vi "TCP数据转换送显示山推.vi"(1 "原始数据":string) -> (0 "数据提取显示":dbl[](array[numeric]))   [LabVIEW 2016]
panel:
  out "*(类型 *) &x":string
  out "截取数据":string
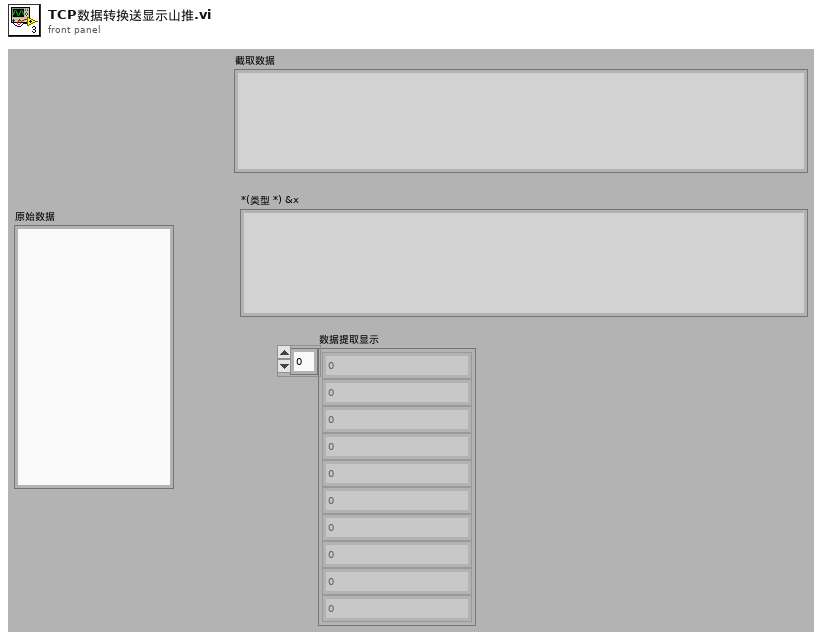
[diagram p1: front panel]
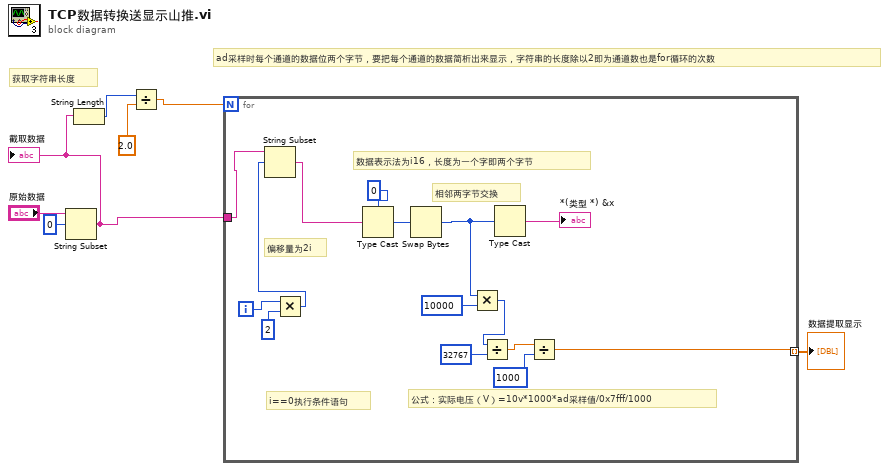
[diagram p0: block diagram]
diagram:
  # "ad采样时每个通道的数据位两个字节，要把每个通道的数据简析出来显示，字符串的长度除以2即为通道数也是for循环的次数"
  # "获取字符串长度"
  n1 = String Subset(string="原始数据", offset (0)=0 ("偏移量(0)")) -> (substring=w5:string)  [unwired: 1 in]
  "截取数据" <- w5
  n2 = String Length(string=w5) -> (length=w3:i32)
  n3 = Divide(x=w3, y=2.0) -> (x/y=w2:dbl)
  n4 = for {
    N: w2 -> [_]
    tunnel: w5 -> [w18]
    tunnel: [w8] -> w1 mode=indexing
    i -> [w15]
    # "公式：实际电压（V）=10v*1000*ad采样值/0x7fff/1000"
    # "i==0执行条件语句"
    # "偏移量为2i"
    # "相邻两字节交换"
    # "数据表示法为i16，长度为一个字即两个字节"
    n5 = Multiply(x=w15, y=2) -> (x*y=w16:i32)
    n6 = String Subset(string=w18, offset (0)=w16) -> (substring=w19:string)  [unwired: 1 in]
    n7 = Type Cast(type=i16 0, x=w19) -> (*(type *) &x=w22:i16)
    n8 = Swap Bytes(anything=w22) -> (byte swapped=w14:i16)
    n9 = Multiply(x=w14, y=10000) -> (x*y=w9:i32)
    n10 = Divide(x=w9, y=i16 32767) -> (x/y=w11:dbl)
    n11 = Type Cast(x=w14) -> (*(type *) &x=→"*(类型 *) &x":string)  [unwired: 1 in]
    n12 = Divide(x=w11, y=i16 1000) -> (x/y=w8:dbl)
  }
  "数据提取显示" <- w1
